vi "Create Tag Path.vi"(8 "error in (no error)":errorcluster, 10 "namespace":string, 11 "tag name":string) -> (0 "error out":errorcluster, 3 "path":string)   [LabVIEW 2017, in "Logger.lvclass"]
uses:
  logger/Logger.lvclass
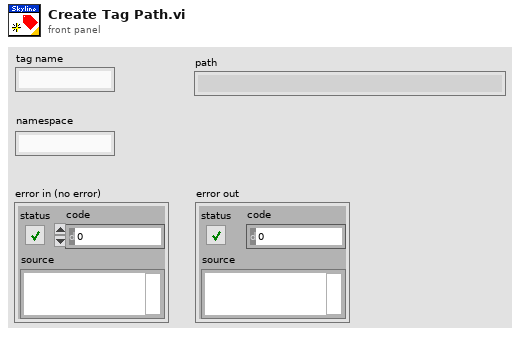
[diagram p1: front panel]
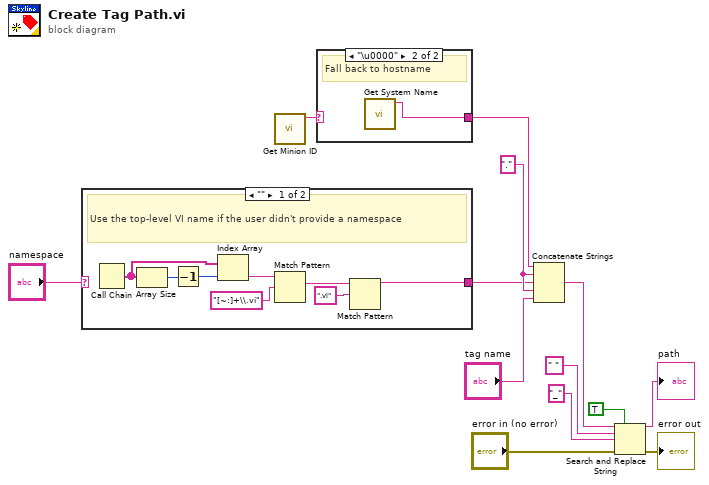
[diagram p0: block diagram]
diagram:
  w4 = "." ("element")
  n1 = case shown="\"\"" "namespace" {
    selector: "namespace" -> [_ w22]
    tunnel: [w14 w22] -> w3
    frame "" {
      # "Use the top-level VI name if the user didn't provide a namespace"
      n2 = Call Chain() -> (call chain=w17:string[])
      n3 = Array Size(array=w17) -> (size(s)=w18:i32)
      n4 = Decrement(x=w18) -> (x-1=w19:i32)
      n5 = Index Array(array=w17, index=w19) -> (element=w20:string)
      n6 = Match Pattern(string=w20, regular expression="[~:]+\\.vi") -> (match substring=w21:string)  [unwired: 1 in, 3 out]
      n7 = Match Pattern(string=w21, regular expression=".vi") -> (before substring=w14:string)  [unwired: 1 in, 3 out]
    }
    frame "valid", Default {
    }
  }
  n8 = call "Get Minion ID.vi"() -> ("minion id"=w2:string)  [unwired: 11 in]
  n9 = case shown="\"\"" w2 {
    selector: w2 -> [w23 _]
    tunnel: [w23 w24] -> w1
    frame Default {
      # "Use the Minion ID if it exists"
    }
    frame "\u0000" {
      # "Fall back to hostname"
      n10 = call "Get System Name.vi"() -> ("name"=w24:string)  [unwired: 11 in]
    }
  }
  n11 = Concatenate Strings(w1, w4, w3, w4, "tag name") -> (w5:string)
  n12 = Search and Replace String(replace all?=TRUE ("replace all? (F)"), input string=w5, search string=" ", replace string="_" ("replace string (\"\")"), error in="error in (no error)") -> (result string=→"path":string, error out=→"error out":errorcluster)  [unwired: 3 in, 2 out]
